vi "capacitance nav xyz.vi"() -> ()   [LabVIEW 2010]
uses:
  <userlib>/Nanonis Prog Interface V5/Nanonis Prog Interface.lvlib
panel:
  in  "Y offset":sgl
  in  "X offset":sgl
  in  "Y sensitivity":sgl=0.001
  in  "X sensitivity":sgl=1.0
  out "Capacitance Z":cluster{"index":i32, sgl}[](graph)
  out "Avg index Z":i32
  out "Avg index Y":i32
  in  "pause":bool
  in  "Delete First Entry":bool
  in  "Time between averages (ms)":u32
  out "Avg index X":i32
  in  "Averages":i32=50
  in  "milliseconds to wait":u32=1000
  in  "stop":bool
  in  "?":bool
  in  "Max Steps":u16=500
  in  "Direction":enum16{"X +", "X -", "Y +", "Y -", "Z +", "Z -"}(ring)
  out "Capacitance Y":cluster{i32, sgl}[](graph)
  in  "Number of Steps":u16=50
  out "Capacitance X":cluster{"index":i32, sgl}[](graph)
  in  "Frequency (Hz)":sgl=261.0
  in  "Amplitude (V)":sgl=350.0
  # "Max Steps On"
  # "Max Steps Off"
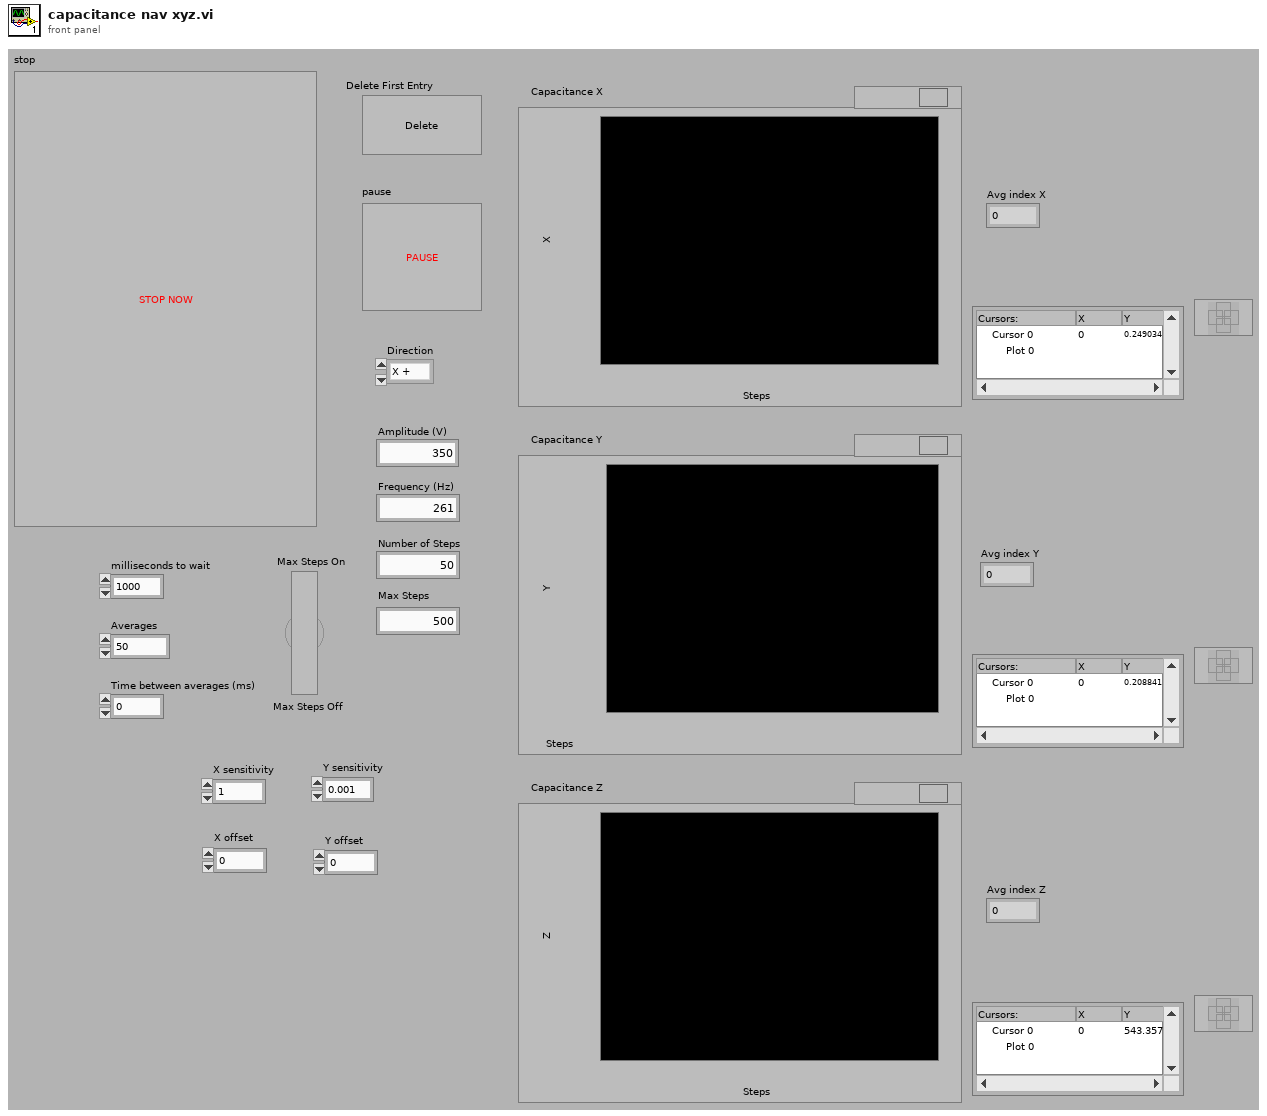
[diagram p1: front panel]
types:
  T1 = enum8{"Group 1", "Group 2", "Group 3", "Group 4", "Group 5", "Group 6"}
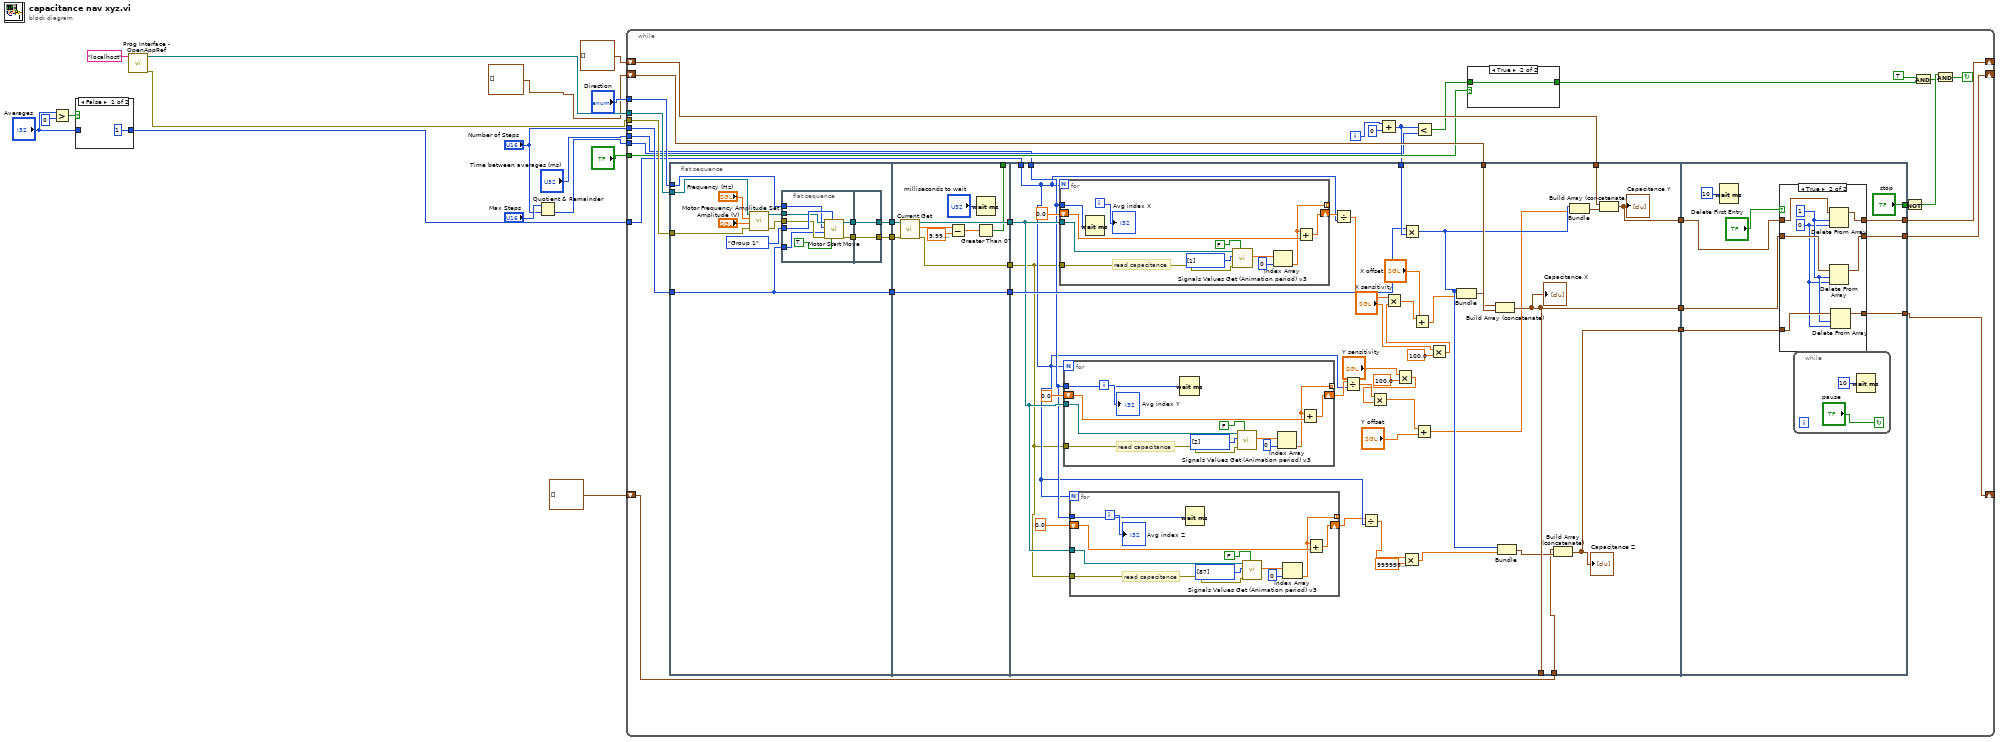
[diagram p0: block diagram]
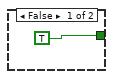
[diagram p3: hidden frame]
diagram:
  n1 = Greater?(x="Averages", y=0) -> (0:w6:bool)
  n2 = case shown="False" w6 {
    tunnel: "Averages" -> [_ w18]
    tunnel: [1 ("Averages") w18] -> w3
    frame False {
    }
    frame True {
    }
  }
  n3 = call <userlib>:"Prog Interface - OpenAppRef.vi"("Machine name (local machine IP)"="localhost" ("machine name (localhost)")) -> ("Error out"=w15:errorcluster, "Application reference"=w14:refnum<vi>)  [unwired: 5 in]
  n4 = Quotient & Remainder(x="Max Steps", y="Number of Steps") -> (floor(x/y)=w9:u16)  [unwired: 1 out]
  n5 = while {
    shift-right: [w22] -> _
    shift-left: cluster{i32, sgl}[] [] -> [w49]
    tunnel: w14 -> [w47]
    tunnel: w15 -> [w46]
    shift-right: [w40] -> _
    shift-left: cluster{i32, sgl}[] [] -> [w39]
    tunnel: "Direction" -> [w38]
    tunnel: "Number of Steps" -> [w37]
    tunnel: w9 -> [w30]
    tunnel: "?" -> [w36]
    tunnel: w3 -> [w25]
    tunnel: "Time between averages (ms)" -> [w24]
    shift-right: [w19] -> _
    shift-left: cluster{i32, sgl}[] [] -> [w21]
    i -> [w33]
    stop <- w27 continue-if-true
    n6 = flat-sequence {
      tunnel: [w55] -> w51
      tunnel: w47 -> [w58]
      tunnel: w46 -> [w61]
      tunnel: [w60] -> w45
      tunnel: [w59] -> w44
      tunnel: w38 -> [w54]
      tunnel: w37 -> [w55]
      tunnel: w51 -> [w86]
      tunnel: [w86] -> w50
      tunnel: w45 -> [w85]
      tunnel: w44 -> [w84]
      tunnel: [w83] -> w43
      tunnel: [w82] -> w42
      tunnel: [w79] -> _
      tunnel: [w115] -> _
      tunnel: w31 -> [w125]
      tunnel: w50 -> [w122]
      tunnel: w49 -> [w123]
      tunnel: w43 -> [w100]
      tunnel: w42 -> [w111]
      tunnel: [w119] -> w41
      tunnel: w39 -> [w120]
      tunnel: w25 -> [w107]
      tunnel: w24 -> [w110]
      tunnel: [w115] -> w23
      tunnel: w21 -> [w102]
      tunnel: [w101] -> w20
      tunnel: w41 -> [w165]
      tunnel: [w164] -> w40
      tunnel: ["stop"] -> w26
      tunnel: [w162] -> w22
      tunnel: w23 -> [w163]
      tunnel: w20 -> [w160]
      tunnel: [w159] -> w19
      frame #0 {
        n7 = call <userlib>:"Motor Frequency Amplitude Set.vi"("Error in (no error)"=w61, "Amplitude (V) (NaN=no change)"="Amplitude (V)", "Frequency (Hz) (NaN=no change)"="Frequency (Hz)", "Application ref in"=w58) -> ("Error out"=w62:errorcluster, "Application ref out"=w63:refnum<vi>)  [unwired: 6 in]
        n8 = flat-sequence {
          tunnel: T1."Group 1" ("Group") -> [w73]
          tunnel: w63 -> [w72]
          tunnel: w62 -> [w71]
          tunnel: w55 -> [w70]
          tunnel: [w69] -> w57
          tunnel: [w68] -> w56
          tunnel: w54 -> [w67]
          tunnel: [w75] -> w59
          tunnel: [w76] -> w60
          tunnel: w57 -> [w76]
          tunnel: w56 -> [w75]
          frame #0 {
            n9 = call <userlib>:"Motor Start Move.vi"("Wait until finished? (F)"=TRUE, "Group"=w73, "Error in (no error)"=w71, "Number of steps"=w70, "Direction"=w67, "Application ref in"=w72) -> ("Error out"=w68:errorcluster, "Application ref out"=w69:refnum<vi>)  [unwired: 3 in]
          }
          frame #1 {
          }
        }
      }
      frame #1 {
        n10 = call <userlib>:"Current Get.vi"("Error in (no error)"=w84, "Application ref in"=w85) -> ("Error out"=w83:errorcluster, "Current (A)"=w81:sgl, "Application ref out"=w82:refnum<vi>)  [unwired: 5 in]
        n11 = Subtract(x=w81, y=sgl 1e-09) -> (x-y=w80:sgl)
        n12 = Greater Than 0?(x=w80) -> (x > 0?=w79:bool)
        n13 = Wait (ms)(milliseconds to wait="milliseconds to wait") -> ()  [unwired: 1 out]
      }
      frame #2 {
        n14 = for {
          N: w107 -> [_]
          tunnel: w100 -> [w155]
          tunnel: w111 -> [w154]
          shift-right: [w152] -> w117
          shift-left: sgl 0.0 ("y") -> [w153]
          tunnel: w110 -> [w150]
          tunnel: [w148] -> _ mode=indexing
          i -> [w151]
          # "read capacitance"
          n15 = Wait (ms)(milliseconds to wait=w150) -> ()  [unwired: 1 out]
          n16 = call <userlib>:"Signals Values Get (Animation period) v3.vi"("Wait for newest data (F=False)"=FALSE, "error in (no error)"=w155, "Signals indexes (0-127)"=i8[] [1], "Application ref in"=w154) -> ("Signals Values"=w156:sgl[])  [unwired: 4 in, 2 out]
          n17 = Index Array(array=w156, index=0) -> (element=w148:sgl)
          n18 = Add(x=w148, y=w153) -> (x+y=w152:sgl)
          "Avg index X" <- w151
        }
        n19 = for {
          N: w107 -> [_]
          tunnel: w100 -> [w144]
          tunnel: w111 -> [w143]
          shift-right: [w141] -> w114
          shift-left: sgl 0.0 ("y") -> [w142]
          tunnel: w110 -> [w139]
          tunnel: [w137] -> _ mode=indexing
          i -> [w140]
          # "read capacitance"
          n20 = Wait (ms)(milliseconds to wait=w139) -> ()  [unwired: 1 out]
          n21 = call <userlib>:"Signals Values Get (Animation period) v3.vi"("Wait for newest data (F=False)"=FALSE, "error in (no error)"=w144, "Signals indexes (0-127)"=i8[] [2], "Application ref in"=w143) -> ("Signals Values"=w145:sgl[])  [unwired: 4 in, 2 out]
          n22 = Index Array(array=w145, index=0) -> (element=w137:sgl)
          n23 = Add(x=w137, y=w142) -> (x+y=w141:sgl)
          "Avg index Y" <- w140
        }
        n24 = for {
          N: w107 -> [_]
          tunnel: w100 -> [w126]
          tunnel: w111 -> [w133]
          shift-right: [w131] -> w103
          shift-left: sgl 0.0 ("y") -> [w132]
          tunnel: w110 -> [w129]
          tunnel: [w127] -> _ mode=indexing
          i -> [w130]
          # "read capacitance"
          n25 = Wait (ms)(milliseconds to wait=w129) -> ()  [unwired: 1 out]
          n26 = call <userlib>:"Signals Values Get (Animation period) v3.vi"("Wait for newest data (F=False)"=FALSE, "error in (no error)"=w126, "Signals indexes (0-127)"=i8[] [87], "Application ref in"=w133) -> ("Signals Values"=w134:sgl[])  [unwired: 4 in, 2 out]
          n27 = Index Array(array=w134, index=0) -> (element=w127:sgl)
          n28 = Add(x=w127, y=w132) -> (x+y=w131:sgl)
          "Avg index Z" <- w130
        }
        n29 = Divide(x=w117, y=w107) -> (x/y=w116:sgl)
        n30 = Divide(x=w114, y=w107) -> (x/y=w99:sgl)
        n31 = Divide(x=w103, y=w107) -> (x/y=w108:sgl)
        n32 = Multiply(x="Y sensitivity", y=sgl 100.0) -> (x*y=w92:sgl)
        n33 = Multiply(x=w99, y=w92) -> (x*y=w98:sgl)
        n34 = Multiply(x=w108, y=sgl 1000000000000.0) -> (x*y=w105:sgl)
        n35 = Multiply(x=w122, y=w125) -> (x*y=w106:i32)
        n36 = Add(x=w98, y="Y offset") -> (x+y=w97:sgl)
        n37 = Multiply(x="X sensitivity", y=sgl 100.0) -> (x*y=w89:sgl)
        n38 = Multiply(x=w116, y=w89) -> (x*y=w96:sgl)
        n39 = Add(x=w96, y="X offset") -> (x+y=w95:sgl)
        n40 = Bundle(w106, w95) -> (w124:cluster{i32, sgl})  [unwired: 1 in]
        n41 = Build Array (concatenate)(w123, w124) -> (w115:cluster{i32, sgl}[])
        "Capacitance X" <- w115
        n42 = Bundle(w106, w105) -> (w104:cluster{i32, sgl})  [unwired: 1 in]
        n43 = Build Array (concatenate)(w102, w104) -> (w101:cluster{i32, sgl}[])
        "Capacitance Z" <- w101
        n44 = Bundle(w106, w97) -> (w121:cluster{i32, sgl})  [unwired: 1 in]
        n45 = Build Array (concatenate)(w120, w121) -> (w119:cluster{i32, sgl}[])
        "Capacitance Y" <- w119
      }
      frame #3 {
        n46 = Wait (ms)(milliseconds to wait=u32 10) -> ()  [unwired: 1 out]
        n47 = case shown="True" "Delete First Entry" {
          tunnel: w165 -> [w172 w180]
          tunnel: [w172 w179] -> w164
          tunnel: w163 -> [w171 w177]
          tunnel: [w171 w178] -> w162
          tunnel: w160 -> [w170 w176]
          tunnel: [w170 w175] -> w159
          frame False {
          }
          frame True {
            w174 = 1 ("length")
            w173 = 0 ("index")
            n48 = Delete From Array(array=w180, length=w174, index=w173) -> (array with subset deleted=w179:cluster{i32, sgl}[])  [unwired: 1 out]
            n49 = Delete From Array(array=w177, length=w174, index=w173) -> (array with subset deleted=w178:cluster{i32, sgl}[])  [unwired: 1 out]
            n50 = Delete From Array(array=w176, length=w174, index=w173) -> (array with subset deleted=w175:cluster{i32, sgl}[])  [unwired: 1 out]
          }
        }
        n51 = while {
          stop <- "pause" continue-if-true
          n52 = Wait (ms)(milliseconds to wait=u32 10) -> ()  [unwired: 1 out]
        }
      }
    }
    n53 = Add(x=w33, y=u16 0) -> (x+y=w31:i32)
    n54 = Less?(x=w31, y=w30) -> (x < y?=w32:bool)
    n55 = case shown="True" w36 {
      tunnel: w32 -> [_ w53]
      tunnel: [TRUE w53] -> w34
      frame False {
      }
      frame True {
      }
    }
    n56 = Not(x=w26) -> (.not. x?=w29:bool)
    n57 = And(x=TRUE, y=w34) -> (x .and. y?=w28:bool)
    n58 = And(x=w29, y=w28) -> (x .and. y?=w27:bool)
  }
